vi "emi_Is Realtime or Embeddedt.vi"(9 "error in (no error)":errorcluster) -> (8 "RT||Emb?":bool, 10 "error out":errorcluster)   [LabVIEW 2011]
doc: "Returns true if vi is running on a realtime or embedded platform. Not including FPGA.\n\nDoes not include error terminals to maximise performance.\n\nSubroutine"
panel:
  # "conditional disable klart raskes.\nFB er ikke langt etter"
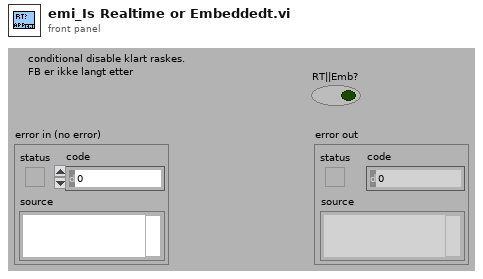
[diagram p1: front panel]
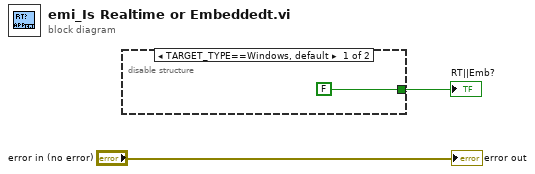
[diagram p0: block diagram]
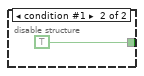
[diagram p2: hidden frame]
diagram:
  n1 = disable-structure shown="TARGET_TYPE==Windows, default" {
    disable-tunnel: [FALSE TRUE ("Boolean")] -> w2
    frame condition #0 (active) {
    }
    frame condition #1 {
    }
  }
  "RT||Emb?" <- w2
  "error out" <- "error in (no error)"
